vi "Create mailbox.vi"(4 "error in (no error)":errorcluster, 5 "max queue size (-1, unlimited)":i32=-1, 7 "name (unnamed)":string) -> (0 "error out":errorcluster, 1 "created new?":bool, 3 "Mailbox ref":T1)   [LabVIEW 2021, in "MatS Libs.lvlib"]
doc: "Wrapped [Obtain queue.vi] to create a mailbox."
uses:
  <userlib>/MatS Libs/MatS Libs.lvlib
  <userlib>/MatS Libs/MatS Mailman/TypeDefs/Mailbox ref.ctl
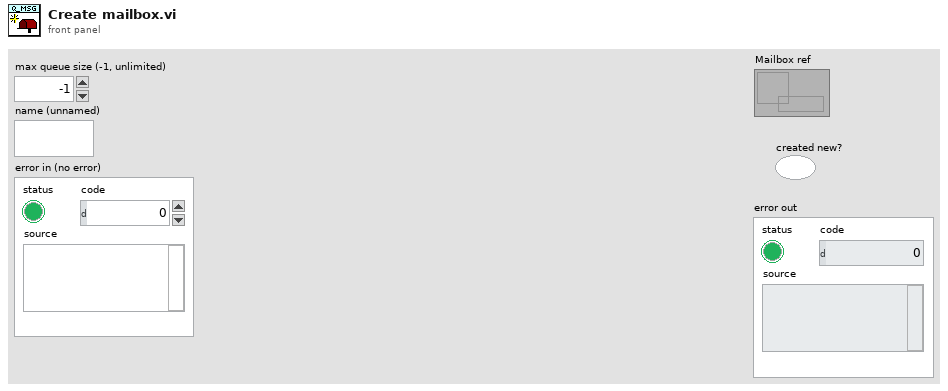
[diagram p1: front panel]
types:
  T1 = typedef "MatS Libs.lvlib/Mailbox ref.ctl" = refnum<queue>
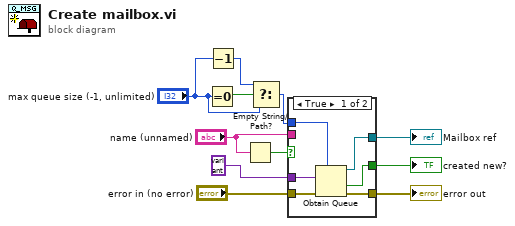
[diagram p0: block diagram]
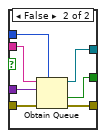
[diagram p2: hidden frame]
diagram:
  n1 = Equal To 0?(x="max queue size (-1, unlimited)") -> (x = 0?=w4:bool)
  n2 = Decrement(x="max queue size (-1, unlimited)") -> (x-1=w3:i32)
  n3 = Empty String/Path?(string/path="name (unnamed)") -> (empty?=w7:bool)
  n4 = Select(t=w3, s=w4, f="max queue size (-1, unlimited)") -> (s? t:f=w1:i32)
  n5 = case shown="True" w7 {
    tunnel: variant -> [w12 w24]
    tunnel: w1 -> [w17 w23]
    tunnel: "name (unnamed)" -> [_ w22]
    tunnel: "error in (no error)" -> [w16 w21]
    tunnel: [w15 w20] -> w9
    tunnel: [w14 w19] -> w8
    tunnel: [w13 w18] -> w5
    frame True {
      n6 = Obtain Queue(max queue size (-1, unlimited)=w17, element data type=w12, error in (no error)=w16) -> (queue out=w13:refnum<queue>, created new?=w14:bool, error out=w15:errorcluster)  [unwired: 2 in]
    }
    frame False {
      n7 = Obtain Queue(max queue size (-1, unlimited)=w23, name (unnamed)=w22, element data type=w24, error in (no error)=w21) -> (queue out=w18:refnum<queue>, created new?=w19:bool, error out=w20:errorcluster)  [unwired: 1 in]
    }
  }
  "error out" <- w9
  "created new?" <- w8
  "Mailbox ref" <- w5
